vi "SngJntArmSim_New.vi"(0 "SimulateGravity":bool, 4 "jKgMetersSquared":dbl, 5 "MaxAngle_Rad":dbl, 6 "ArmLength_Meters":dbl, 7 "MinAngle_Rad":dbl, 8 "MeasurementStdDev":T1, 9 "ArmMass_Kg":dbl, 10 "Gearing":dbl=1.0, 11 "GearBox":T2 {"Kt_NMPerAmp" format="%13.5p"; "Kv_RadPerSecPerVolt" format="%13.5p"; "R_Ohms" format="%13.5p"; "FreeSpeed_RadPerSec" format="%13.5p"; "FreeCurrent_Amps" format="%13.5p"; "StallCurrent_Amps" format="%13.5p"; "StallTorque_NM" format="%13.5p"; "nominalVoltage_Volts" format="%13.5p"}) -> (3 "SingleJointArmSim":T3 {"GearBox"."Kt_NMPerAmp" format="%13.5p"; "GearBox"."Kv_RadPerSecPerVolt" format="%13.5p"; "GearBox"."R_Ohms" format="%13.5p"; "GearBox"."FreeSpeed_RadPerSec" format="%13.5p"; "GearBox"."FreeCurrent_Amps" format="%13.5p"; "GearBox"."StallCurrent_Amps" format="%13.5p"; "GearBox"."StallTorque_NM" format="%13.5p"; "GearBox"."nominalVoltage_Volts" format="%13.5p"})   [LabVIEW 2019, in "Trajectory_Library.lvlib"]
doc: "Creates a new LINEAR SYSTEM data cluster with the specified values. \n\n\nInputs: \n - XXX -- XXX.\n\nOutputs:\n - XXX -- XXX."
uses:
  Trajectory_Library.lvlib
  <vilib>/Analysis/Matrix/Datatypes/RealMatrix.ctl
  <vilib>/Analysis/Matrix/NI_Matrix.lvlib
  LINEAR_SYSTEM.ctl
  DCMOTOR.CTL
  LINEAR_SYSTEM_SIM.ctl
  SINGLE_JOINT_ARM_SIM.ctl
panel:
  # "<1, 1>"
  # "<States, 1>"
  # "<Outputs, 1>"
  # "<Inputs, 1>"
  # "<Outputs, 1>"
  # "<States,States>"
  # "<States,Inputs>"
  # "<Outputs,States>"
  # "<Outputs,Inputs>"
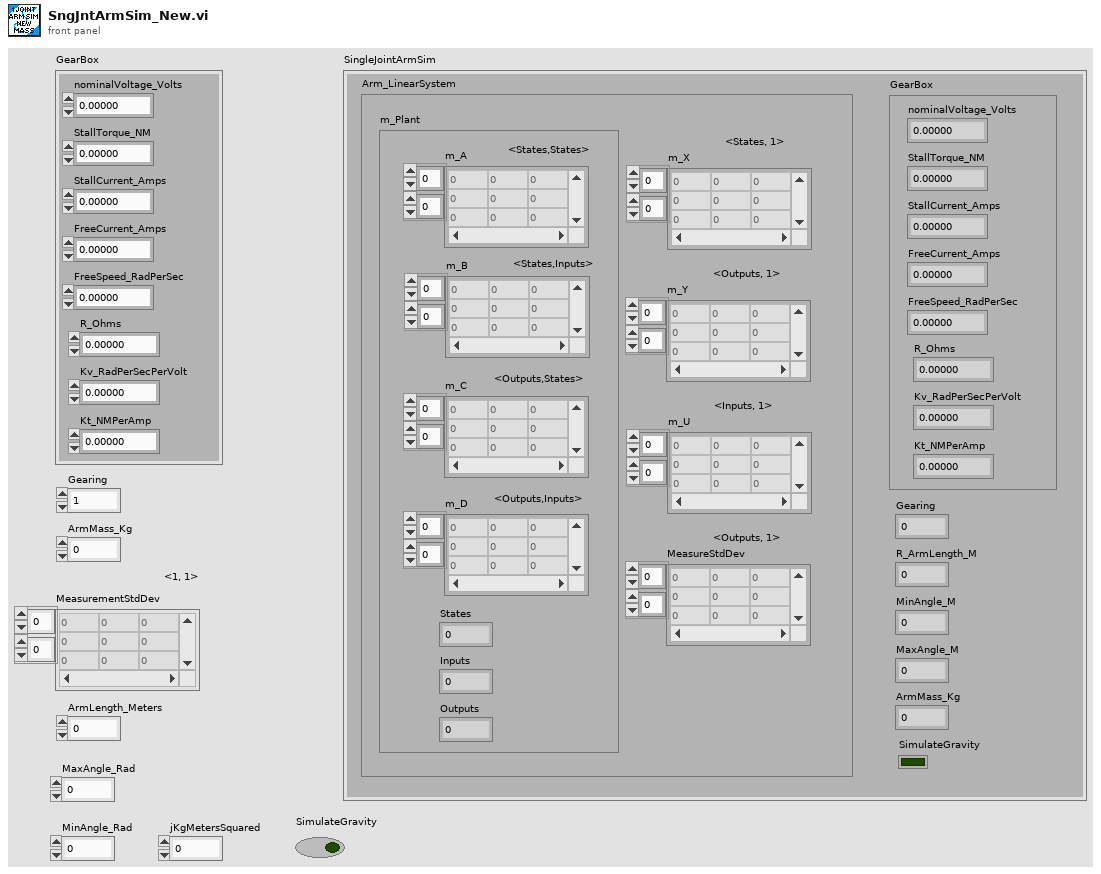
[diagram p1: front panel]
types:
  T1 = typedef "NI_Matrix.lvlib/RealMatrix.ctl" = dbl[][]
  T2 = typedef "Trajectory_Library.lvlib/DCMOTOR.CTL" = cluster{"nominalVoltage_Volts":dbl, "StallTorque_NM":dbl, "StallCurrent_Amps":dbl, "FreeCurrent_Amps":dbl, "FreeSpeed_RadPerSec":dbl, "R_Ohms":dbl, "Kv_RadPerSecPerVolt":dbl, "Kt_NMPerAmp":dbl}
  T3 = typedef "Trajectory_Library.lvlib/SINGLE_JOINT_ARM_SIM.ctl" = cluster{"Arm_LinearSystem":T4, "GearBox":T2, "Gearing":dbl, "R_ArmLength_M":dbl, "MinAngle_M":dbl, "MaxAngle_M":dbl, "ArmMass_Kg":dbl, "SimulateGravity":bool}
  T4 = typedef "Trajectory_Library.lvlib/LINEAR_SYSTEM_SIM.ctl" = cluster{"m_Plant":T5, "m_X":T1, "m_Y":T1, "m_U":T1, "MeasureStdDev":T1}
  T5 = typedef "Trajectory_Library.lvlib/LINEAR_SYSTEM.ctl" = cluster{"m_A":T1, "m_B":T1, "m_C":T1, "m_D":T1, "States":i32, "Inputs":i32, "Outputs":i32}
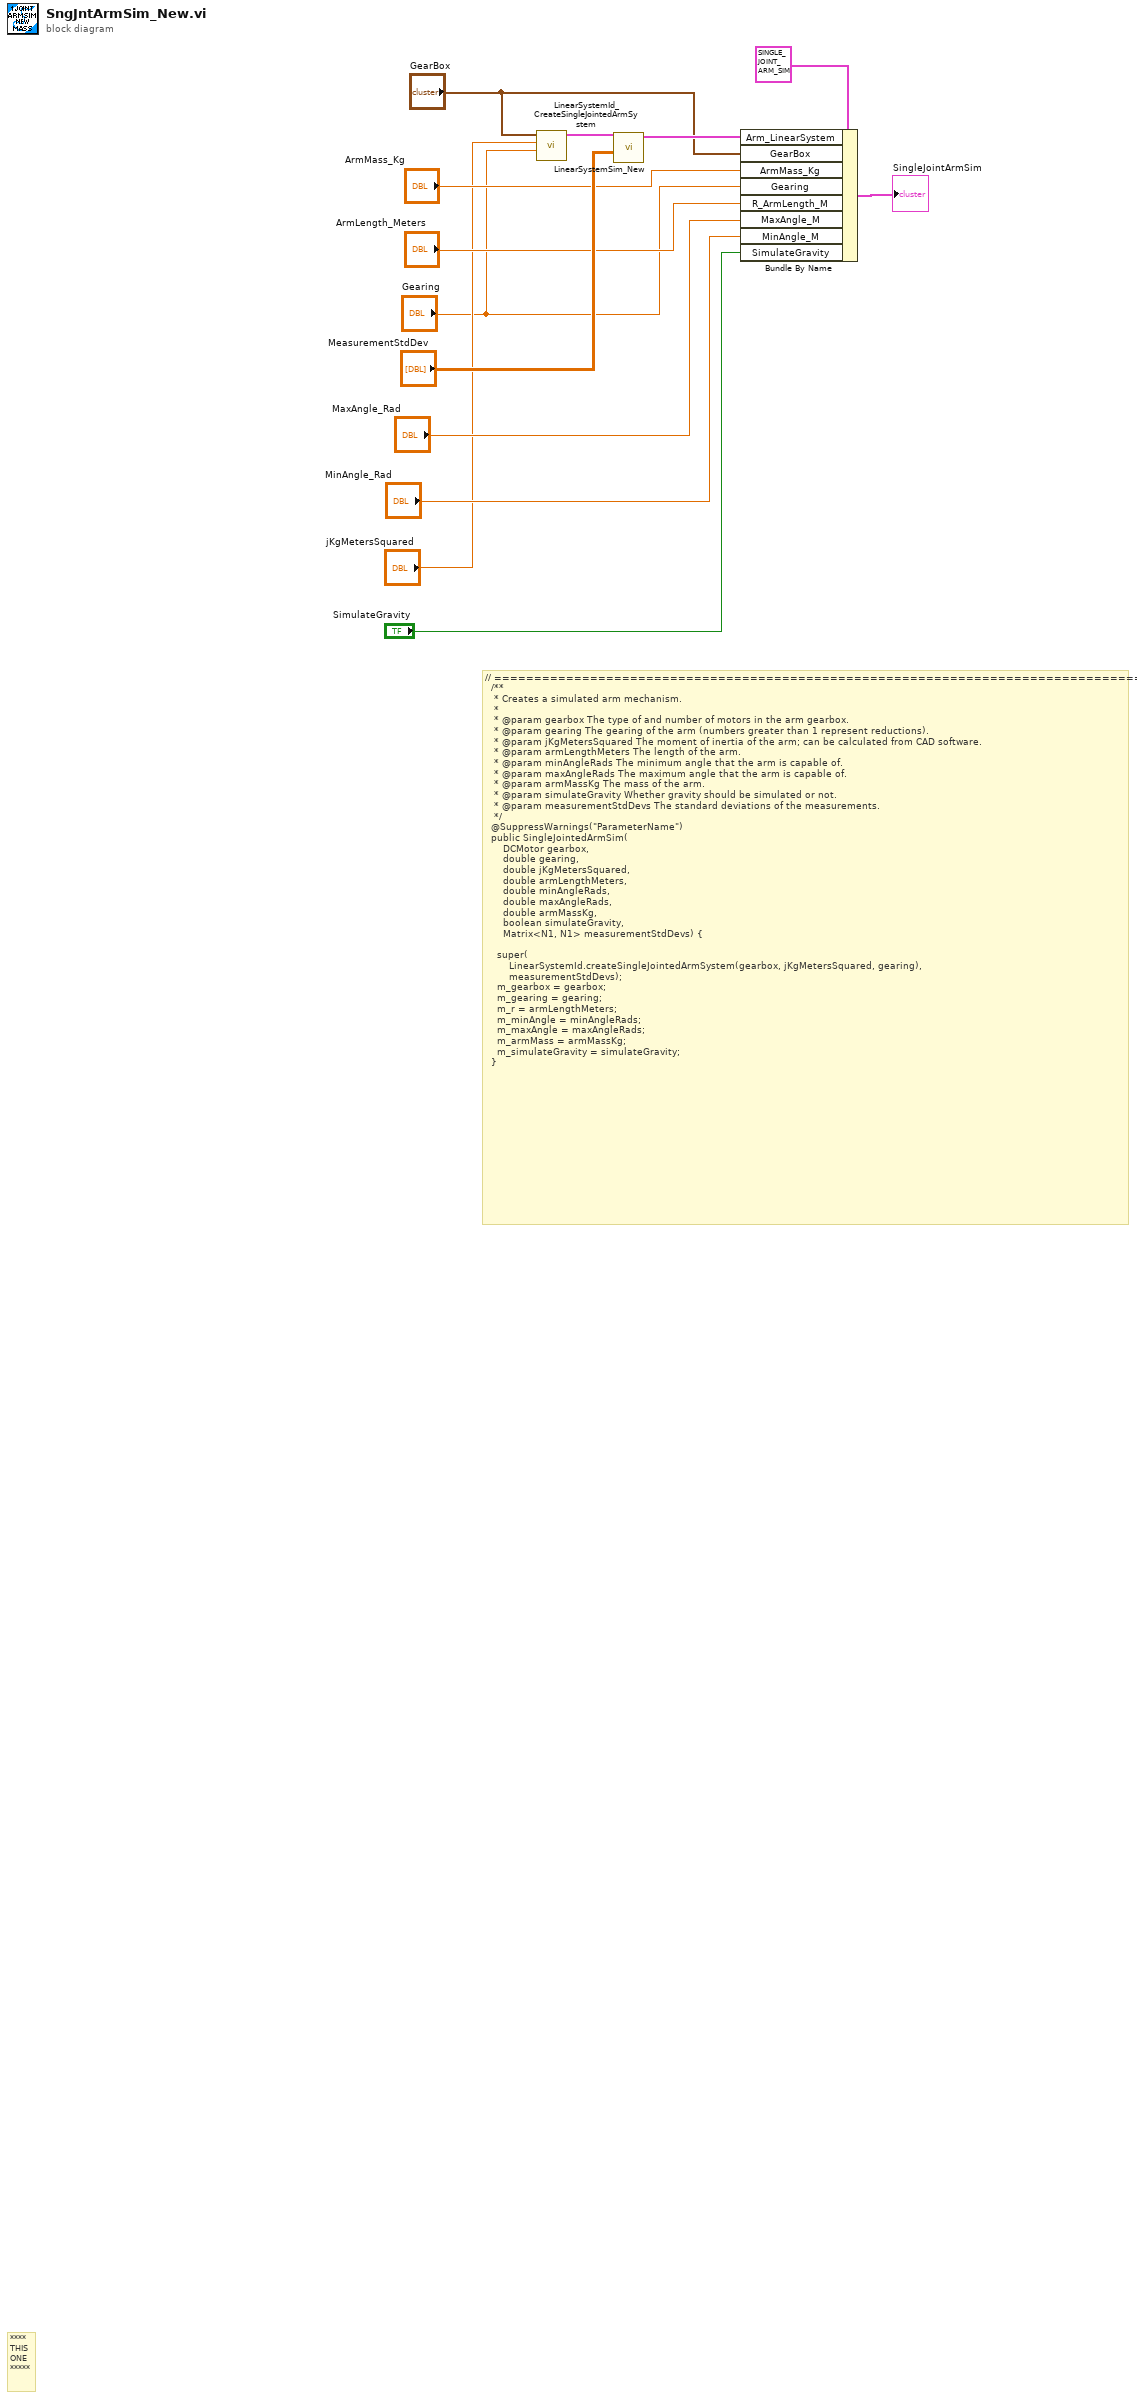
[diagram p0: block diagram]
diagram:
  # "// =================================================================================\n  /**\n   * Creates a simulated arm mechanism.\n   *\n   * @param gearbox The type of and number of motors in the arm gearbox.\n   * @param gearing The gearing of the arm (numbers greater than 1 represent reductions).\n   * @param jKgMetersSquared The moment of inertia of the arm; can be calculated from CAD software.\n   * @param armLengthMeters The length of the arm.\n   * @param minAngleRads The minimum angle that the arm is capable of.\n   * @param maxAngleRads The maximum angle that the arm is capable of.\n   * @param armMassKg The mass of the arm.\n   * @param simulateGravity Whether gravity should be simulated or not.\n   * @param measurementStdDevs The standard deviations of the measurements.\n   */\n  @SuppressWarnings(\"ParameterName\")\n  public SingleJointedArmSim(\n      DCMotor gearbox,\n      double gearing,\n      double jKgMetersSquared,\n      double armLengthMeters,\n      double minAngleRads,\n      double maxAngleRads,\n      double armMassKg,\n      boolean simulateGravity,\n      Matrix<N1, N1> measurementStdDevs) {\n\n    super(\n        LinearSystemId.createSingleJointedArmSystem(gearbox, jKgMetersSquared, gearing),\n        measurementStdDevs);\n    m_gearbox = gearbox;\n    m_gearing = gearing;\n    m_r = armLengthMeters;\n    m_minAngle = minAngleRads;\n    m_maxAngle = maxAngleRads;\n    m_armMass = armMassKg;\n    m_simulateGravity = simulateGravity;\n  }"
  # "****\nTHIS\nONE\n*****"
  n1 = call "LinearSystemId_CreateSingleJointedArmSystem.vi"("G"="Gearing", "jKgSquaredMeters"="jKgMetersSquared", "DCMOTOR"="GearBox") -> ("Linearsystem"=w5:T5)  [unwired: 8 in]
  n2 = call "LinearSystemSim_New.vi"("MeasurementStdDev"="MeasurementStdDev", "System"=w5) -> ("LinearSystemSim"=w11:T4)  [unwired: 9 in]
  n3 = Bundle By Name(cluster=T3 {"Arm_LinearSystem"={"m_Plant"={"m_A"=[], "m_B"=[], "m_C"=[], "m_D"=[], "States"=0, "Inputs"=0, "Outputs"=0}, "m_X"=[], "m_Y"=[], "m_U"=[], "MeasureStdDev"=[]}, "GearBox"={"nominalVoltage_Volts"=0.0, "StallTorque_NM"=0.0, "StallCurrent_Amps"=0.0, "FreeCurrent_Amps"=0.0, "FreeSpeed_RadPerSec"=0.0, "R_Ohms"=0.0, "Kv_RadPerSecPerVolt"=0.0, "Kt_NMPerAmp"=0.0}, "Gearing"=0.0, "R_ArmLength_M"=0.0, "MinAngle_M"=0.0, "MaxAngle_M"=0.0, "ArmMass_Kg"=0.0, "SimulateGravity"=FALSE} ("SINGLE_JOINT_ARM_SIM"), "Arm_LinearSystem"=w11, "GearBox"="GearBox", "ArmMass_Kg"="ArmMass_Kg", "Gearing"="Gearing", "R_ArmLength_M"="ArmLength_Meters", "MaxAngle_M"="MaxAngle_Rad", "MinAngle_M"="MinAngle_Rad", "SimulateGravity"="SimulateGravity") -> (→"SingleJointArmSim":T3)
